vi "Com_SECS Equipment _Data Message_List.vi"(7 "Parent Index":i32=-1, 8 "error in":errorcluster, 11 "Message Data In":T1[](array[typedef])) -> (0 "error out":errorcluster, 2 "Index":i32, 3 "Message Data Out":T1[](array[typedef]))   [LabVIEW 2016]
uses:
  Data Def/Com_SECS Equipment _Message Data.ctl
  Data Def/Com_SECS Equipment _Data Item Format.ctl
  Data Def/Com_SECS Equipment _Format Code.ctl
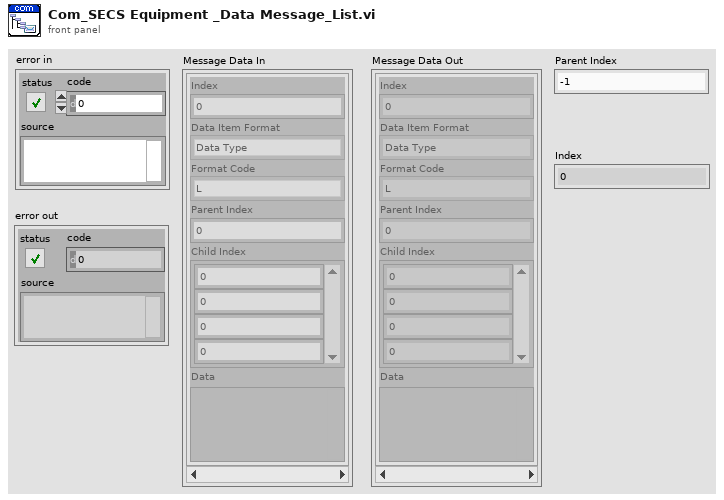
[diagram p1: front panel]
types:
  T1 = typedef "Com_SECS Equipment _Message Data.ctl" = cluster{"Index":i32, "Data Item Format":T2, "Format Code":T3, "Parent Index":i32, "Child Index":i32[], "Data":variant}
  T2 = typedef "Com_SECS Equipment _Data Item Format.ctl" = enum16{"Data Type", "Value"}
  T3 = typedef "Com_SECS Equipment _Format Code.ctl" = enum16{"L", "A", "B", "Boolean", "J", "I1", "I2", "I4", "I8", "U1", "U2", "U4", "U8", "F4", "F8", "Char"}
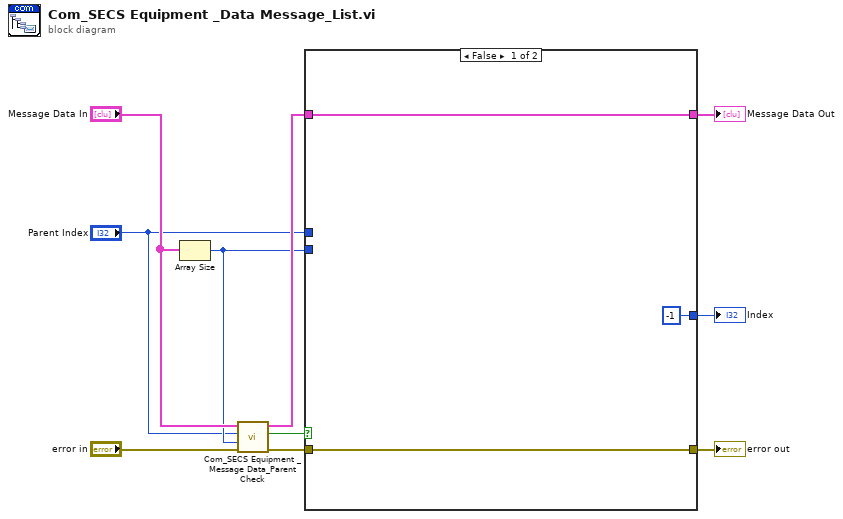
[diagram p0: block diagram]
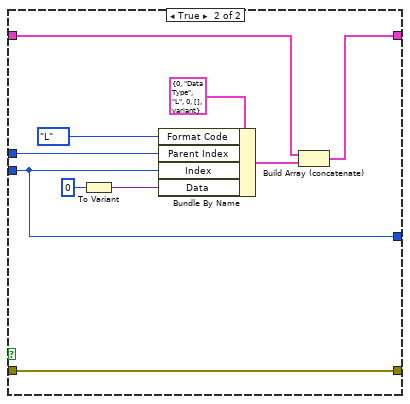
[diagram p2: hidden frame]
diagram:
  n1 = Array Size(array="Message Data In") -> (size(s)=w5:i32)
  n2 = call "Com_SECS Equipment _Message Data_Parent Check.vi"("error in"="error in", "Message Index"=w5, "Parent Index"="Parent Index", "Message Data In"="Message Data In") -> ("error out"=w8:errorcluster, "OK?"=w9:bool, "Message Data Out"=w6:T1[])  [unwired: 5 in]
  n3 = case shown="False" w9 {
    tunnel: w8 -> [w12 w17]
    tunnel: w6 -> [w13 w19]
    tunnel: [w13 w18] -> w4
    tunnel: "Parent Index" -> [_ w20]
    tunnel: w5 -> [_ w14]
    tunnel: [w12 w17] -> w3
    tunnel: [-1 w14] -> w2
    frame False {
    }
    frame True {
      n4 = To Variant(anything=0) -> (Variant=w21:variant)
      n5 = Bundle By Name(cluster=T1 {"Index"=0, "Data Item Format"=enum."Data Type", "Format Code"=enum."L", "Parent Index"=0, "Child Index"=[], "Data"=variant} ("Message Data"), "Format Code"=Com_SECS_Equipment__Format_Code."L", "Parent Index"=w20, "Index"=w14, "Data"=w21) -> (w15:T1)
      n6 = Build Array (concatenate)(w19, w15) -> (w18:T1[])
    }
  }
  "error out" <- w3
  "Message Data Out" <- w4
  "Index" <- w2
